vi "Create RPC Method.vi"(8 "error in (no error)":errorcluster, 10 "rpc method parameters":T1, 11 "server class in":refnum<vi>) -> (0 "error out":errorcluster, 2 "newly created ?":bool, 3 "server class out":refnum<vi>)   [LabVIEW 2019, in "gRPC Template Creation Utility.lvlib"]
uses:
  gRPC Template Creation Utility.lvlib
  TypeDefs/RPC Method Parameters.ctl
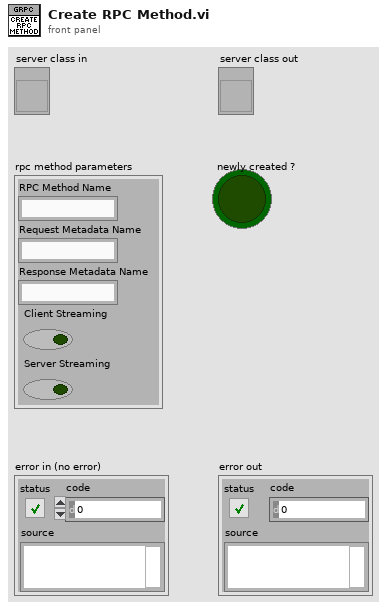
[diagram p1: front panel]
types:
  T1 = typedef "gRPC Template Creation Utility.lvlib/RPC Method Parameters.ctl" = cluster{"RPC Method Name":string, "Request Metadata Name":string, "Response Metadata Name":string, "Client Streaming":bool, "Server Streaming":bool}
  T2 = enum32{"invalid VI type", "Standard VI", "Control VI", "Global VI", "Polymorphic VI", "Configuration VI", "SubSystem", "Facade VI", "Method VI"}
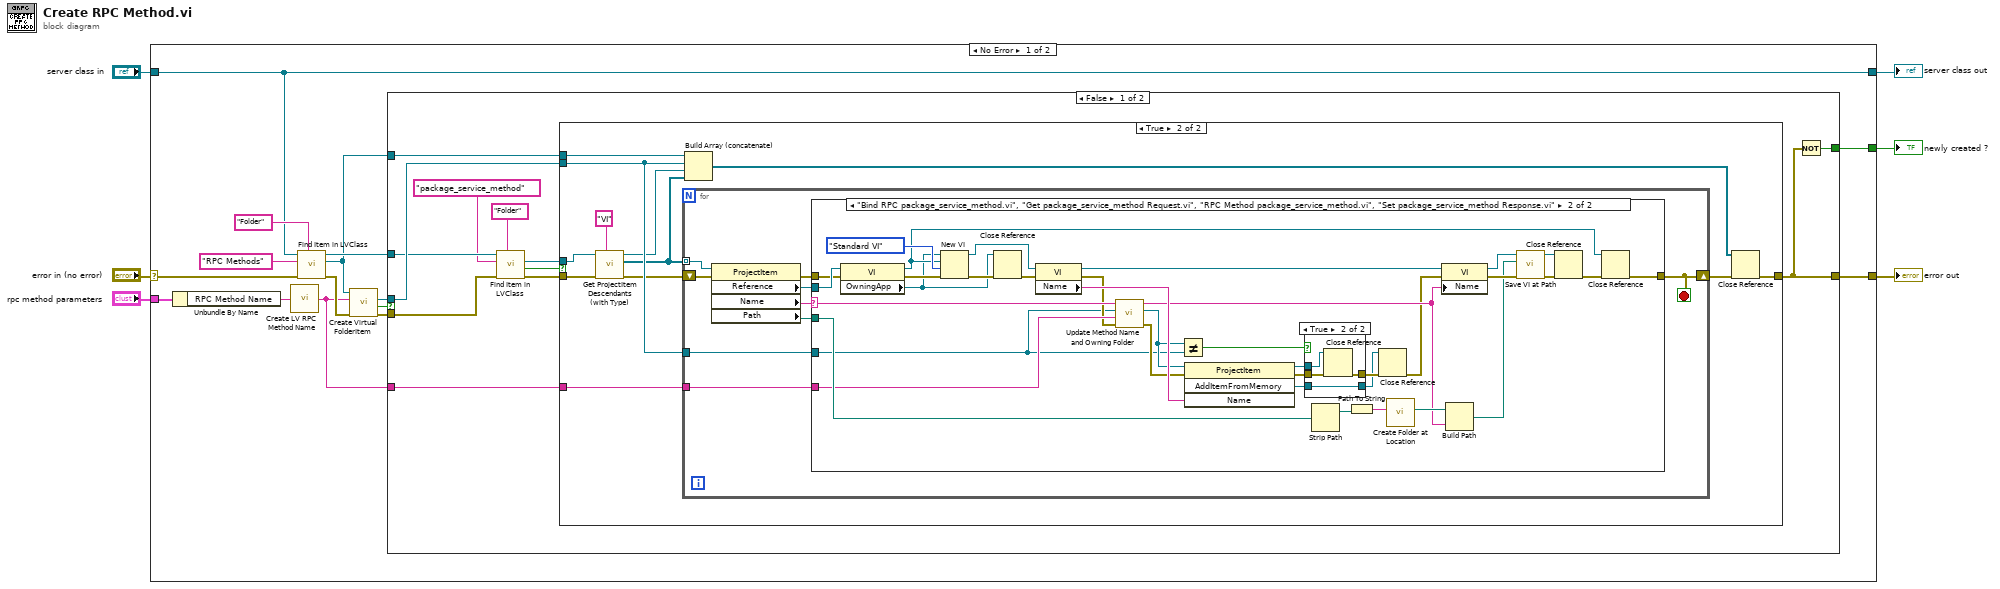
[diagram p0: block diagram]
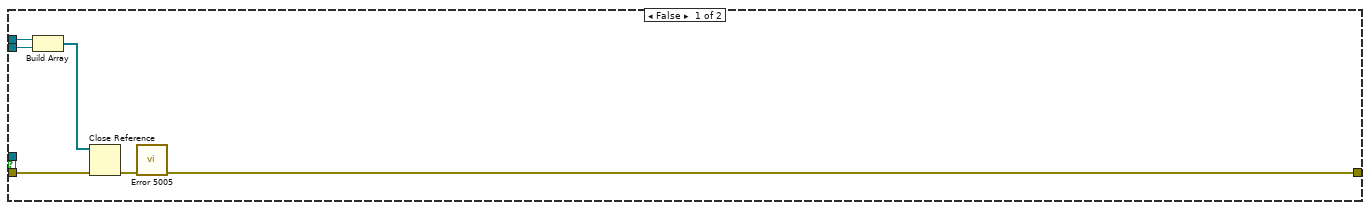
[diagram p2: hidden frame]
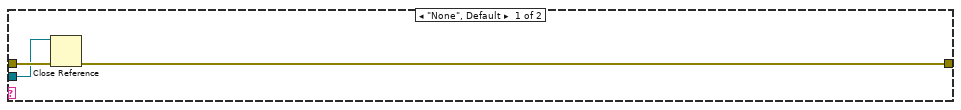
[diagram p3: hidden frame]
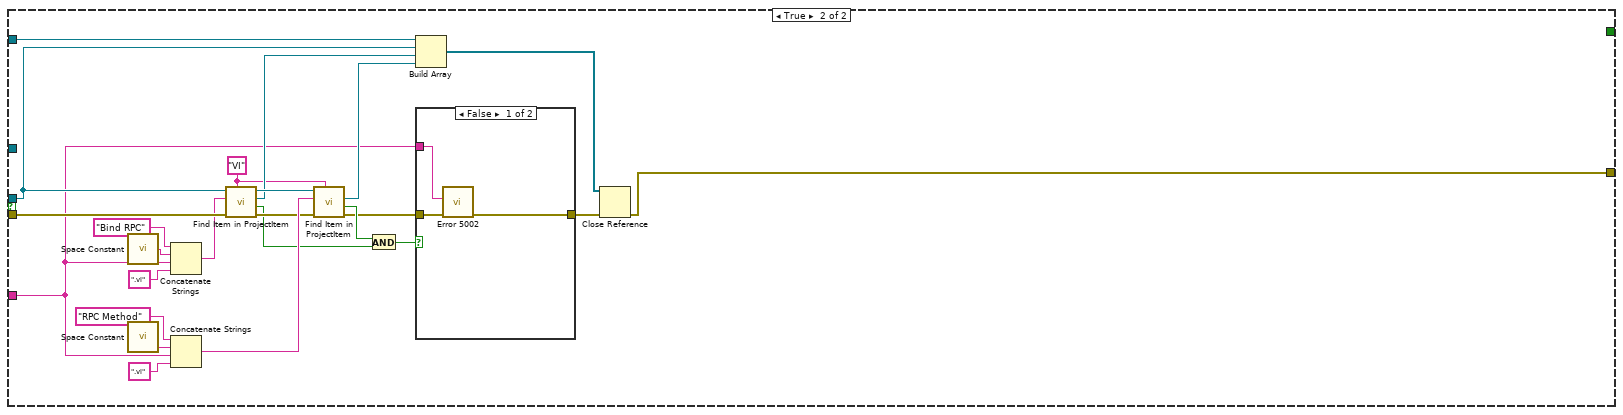
[diagram p5: hidden frame]
diagram:
  n1 = case shown="No Error" "error in (no error)" {
    selector: "error in (no error)" -> [w12 w135]
    tunnel: "server class in" -> [w11 w134]
    tunnel: [w17 w135] -> w5
    tunnel: [w11 w134] -> w3
    tunnel: [w10 _] -> w2
    tunnel: "rpc method parameters" -> [w9 _]
    frame No Error {
      n2 = Unbundle By Name(w9) -> ("RPC Method Name"=w8:string)
      n3 = call "Create LV RPC Method Name.vi"("Proto Parser RPC Method Name in"=w8) -> ("LV RPC Method Name out"=w7:string)
      n4 = call "Find Item in LVClass.vi"("Item Type"="Folder", "error in (no error)"=w12, "Item Name"="RPC Methods", "Class Item in"=w11) -> ("error out"=w16:errorcluster, "Project Item (Class Item)"=w14:refnum<vi>, "Class Item out"=w18:refnum<vi>)  [unwired: 4 in, 1 out]
      n5 = call "Create Virtual FolderItem.vi"("error in (no error)"=w16, "Folder Name"=w7, "ProjectItem in"=w14) -> ("error out"=w15:errorcluster, "Already exists?"=w21:bool, "FolderItem reference out"=w13:refnum<vi>)  [unwired: 5 in, 1 out]
      n6 = case shown="False" w21 {
        tunnel: w13 -> [w33 w114]
        tunnel: w14 -> [w32 w115]
        tunnel: w15 -> [w31 w129]
        tunnel: [w26 w106] -> w17
        tunnel: w18 -> [w30 _]
        tunnel: w7 -> [w27 w110]
        tunnel: [w25 _] -> w10
        frame False {
          n7 = call "Find Item in LVClass.vi"("Item Type"="Folder", "error in (no error)"=w31, "Item Name"="package_service_method", "Class Item in"=w30) -> ("error out"=w23:errorcluster, "Found?"=w22:bool, "Project Item (Class Item)"=w24:refnum<vi>)  [unwired: 4 in, 1 out]
          n8 = case shown="True" w22 {
            tunnel: w33 -> [w37 w51]
            tunnel: w32 -> [w38 w50]
            tunnel: w27 -> [_ w48]
            tunnel: [w39 w47] -> w26
            tunnel: w24 -> [_ w46]
            tunnel: w23 -> [w36 w45]
            frame False {
              n9 = Build Array(w38, w37) -> (w35:refnum<vi>[])
              n10 = Close Reference(reference=w35, error in (no error)=w36) -> (error out=w34:errorcluster)
              n11 = call "Error 5005.vi"("error in (no error)"=w34) -> ("error out"=w39:errorcluster)  [unwired: 10 in]
            }
            frame True {
              n12 = call "Get ProjectItem Descendants (with Type).vi"("Type"="VI", "error in (no error)"=w45, "ProjectItem in"=w46) -> ("error out"=w41:errorcluster, "All Descendents"=w42:refnum<vi>[], "ProjectItem out"=w43:refnum<vi>)  [unwired: 6 in]
              n13 = for {
                tunnel: w42 -> [w60] mode=indexing
                tunnel: w51 -> [w54]
                tunnel: w48 -> [w55]
                shift-right: [w52] -> w40
                shift-left: w41 -> [w59]
                stop <- w52 stop-if-true
                n14 = property class="ProjectItem"(reference=w60, error in=w59) -> (error out=w53:errorcluster, "Reference"=w57:refnum<vi>, "Name"=w58:string, "Path"=w56:path)  [unwired: 1 out]
                n15 = case shown="\"Bind RPC package_service_method.vi\", \"Get package_service_method Request.vi\", \"RPC Method package_service_method.vi\", \"Set package_service_method Response.vi\"" w58 {
                  selector: w58 -> [_ w87]
                  tunnel: w57 -> [w61 w84]
                  tunnel: w56 -> [_ w89]
                  tunnel: w55 -> [_ w85]
                  tunnel: w54 -> [_ w71]
                  tunnel: w53 -> [w63 w83]
                  tunnel: [w62 w77] -> w52
                  frame "None", Default {
                    n16 = Close Reference(reference=w61, error in (no error)=w63) -> (error out=w62:errorcluster)
                  }
                  frame "Bind RPC package_service_method.vi", "Get package_service_method Request.vi", "RPC Method package_service_method.vi", "Set package_service_method Response.vi" {
                    n17 = property class="VI"(reference=w84, error in=w83) -> (reference out=w76:refnum<vi>, error out=w82:errorcluster, "OwningApp"=w64:refnum<vi>)
                    n18 = New VI(8:w82, 9:T2."Standard VI" ("vi type (standard vi)"), 10:w76, 11:w64) -> (0:w67:errorcluster, 3:w66:refnum<vi>)  [unwired: 3 out]
                    n19 = Close Reference(reference=w64, error in (no error)=w67) -> (error out=w65:errorcluster)
                    n20 = property class="VI"(reference=w66, error in=w65) -> (reference out=w97:refnum<vi>, error out=w81:errorcluster, "Name"=w99:string)
                    n21 = call "Update Method Name and Owning Folder.vi"("error in"=w81, "rpc method name"=w85, "rpc method folder"=w71, "original vi name"=w87) -> ("error out"=w80:errorcluster, "owning folder"=w72:refnum<vi>, "new vi name"=w86:string)  [unwired: 5 in]
                    n22 = Not Equal?(x=w72, y=w71) -> (x != y?=w70:bool)
                    n23 = invoke class="ProjectItem" method="AddItemFromMemory"(reference=w72, error in=w80, "Name"=w99) -> (reference out=w73:refnum<vi>, error out=w75:errorcluster, "AddItemFromMemory"=w69:refnum<vi>)  [unwired: 1 in, 1 out]
                    n24 = case shown="True" w70 {
                      tunnel: w75 -> [w101 w105]
                      tunnel: [w101 w104] -> w74
                      tunnel: w73 -> [_ w103]
                      tunnel: w69 -> [w100 w102]
                      tunnel: [w100 w102] -> w68
                      frame False {
                      }
                      frame True {
                        n25 = Close Reference(reference=w103, error in (no error)=w105) -> (error out=w104:errorcluster)
                      }
                    }
                    n26 = Strip Path(path=w89) -> (stripped path=w88:path)  [unwired: 1 out]
                    n27 = Path To String(path=w88) -> (string=w94:string)
                    n28 = Close Reference(reference=w68, error in (no error)=w74) -> (error out=w79:errorcluster)
                    n29 = call "Create Folder at Location.vi"("Path"=w94) -> ("Full path out"=w93:path)  [unwired: 8 in, 2 out]
                    n30 = property class="VI"(reference=w97, error in=w79, "Name"=w86) -> (reference out=w96:refnum<vi>, error out=w95:errorcluster)
                    n31 = Build Path(base path=w93, name or relative path=w86) -> (appended path=w92:path)
                    n32 = call "Save VI at Path.vi"("error in (no error)"=w95, "Path"=w92, "VI in"=w96) -> ("error out"=w91:errorcluster, "VI out"=w90:refnum<vi>)  [unwired: 6 in, 1 out]
                    n33 = Close Reference(reference=w90, error in (no error)=w91) -> (error out=w78:errorcluster)
                    n34 = Close Reference(reference=w76, error in (no error)=w78) -> (error out=w77:errorcluster)
                  }
                }
              }
              n35 = Build Array (concatenate)(w50, w51, w43, w42) -> (w49:refnum<vi>[])
              n36 = Close Reference(reference=w49, error in (no error)=w40) -> (error out=w47:errorcluster)
            }
          }
          n37 = Not(x=w26) -> (.not. x?=w25:bool)
        }
        frame True {
          w108 = "VI" ("Type")
          n38 = call <vilib>:"Space Constant.vi"() -> ("String"=w123:string)
          n39 = call <vilib>:"Space Constant.vi"() -> ("String"=w122:string)
          n40 = Concatenate Strings("Bind RPC" ("string"), w123, w110, ".vi" ("string")) -> (w126:string)
          n41 = Concatenate Strings("RPC Method" ("string"), w122, w110, ".vi" ("string")) -> (w120:string)
          n42 = call "Find Item in ProjectItem.vi"("Item Type"=w108, "error in (no error)"=w129, "Name"=w126, "ProjectItem in"=w114) -> ("error out"=w119:errorcluster, "Found ?"=w118:bool, "Item Refnum out"=w113:refnum<vi>, "ProjectItem out"=w128:refnum<vi>)  [unwired: 4 in]
          n43 = call "Find Item in ProjectItem.vi"("Item Type"=w108, "error in (no error)"=w119, "Name"=w120, "ProjectItem in"=w128) -> ("error out"=w111:errorcluster, "Found ?"=w117:bool, "Item Refnum out"=w112:refnum<vi>)  [unwired: 4 in, 1 out]
          n44 = And(x=w117, y=w118) -> (x .and. y?=w116:bool)
          n45 = Build Array(w115, w114, w113, w112) -> (w109:refnum<vi>[])
          n46 = case shown="False" w116 {
            tunnel: w111 -> [w132 w133]
            tunnel: w110 -> [w130 _]
            tunnel: [w131 w133] -> w107
            frame False {
              n47 = call "Error 5002.vi"("error in (no error)"=w132, "Method Name"=w130) -> ("error out"=w131:errorcluster)  [unwired: 9 in]
            }
            frame True {
            }
          }
          n48 = Close Reference(reference=w109, error in (no error)=w107) -> (error out=w106:errorcluster)
        }
      }
    }
    frame Error {
    }
  }
  "error out" <- w5
  "server class out" <- w3
  "newly created ?" <- w2
